vi "TurboState.vi"(11 "Numeric":dbl) -> (3 "String":string)   [LabVIEW 2015]
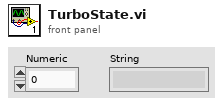
[diagram p1: front panel]
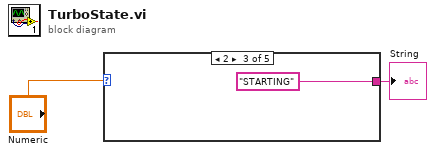
[diagram p0: block diagram]
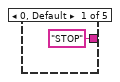
[diagram p2: hidden frame]
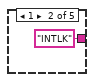
[diagram p3: hidden frame]
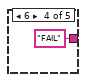
[diagram p4: hidden frame]
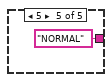
[diagram p5: hidden frame]
diagram:
  n1 = case shown="2" "Numeric" {
    tunnel: ["STOP" "INTLK" "STARTING" "FAIL" "NORMAL"] -> w2
    frame 0, Default {
    }
    frame 1 {
    }
    frame 2 {
    }
    frame 6 {
    }
    frame 5 {
    }
  }
  "String" <- w2
